vi "Initialize board layout.vi"() -> (0 "Initialized board":refnum<class "Board.lvclass">)   [LabVIEW 2016, in "Chesslib.lvlib" / "Position.lvclass"]
uses:
  Position.lvclass
  Board/Board.lvclass
  typedef/Square.ctl
  typedef/File.ctl
  typedef/Rank.ctl
  typedef/Piece.ctl
  typedef/Color.ctl
  typedef/Piece type.ctl
  Chesslib.lvlib
  Pieces/Piece/Piece.lvclass
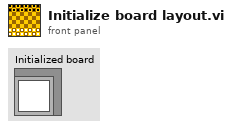
[diagram p1: front panel]
types:
  T1 = typedef "Chesslib.lvlib/Square.ctl" = cluster{"File":T2, "Rank":T3}
  T2 = typedef "Chesslib.lvlib/File.ctl" = enum8{"a", "b", "c", "d", "e", "f", "g", "h"}
  T3 = typedef "Chesslib.lvlib/Rank.ctl" = enum8{"1", "2", "3", "4", "5", "6", "7", "8"}
  T4 = typedef "Chesslib.lvlib/Piece.ctl" = cluster{"Color":T5, "Type":T6}
  T5 = typedef "Chesslib.lvlib/Color.ctl" = enum16{"White", "Black"}
  T6 = typedef "Chesslib.lvlib/Piece type.ctl" = enum16{"Pawn", "Bishop", "Knight", "Rook", "Queen", "King"}
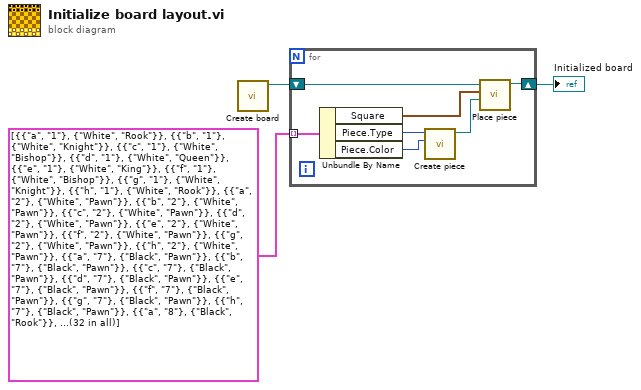
[diagram p0: block diagram]
diagram:
  n1 = call "Create board.vi"() -> ("Empty board"=w2:refnum<class "Board.lvclass">)  [unwired: 11 in]
  n2 = for {
    tunnel: cluster{"Square":T1, "Piece":T4}[] [{"Square"={"File"=enum."a", "Rank"=enum."1"}, "Piece"={"Color"=enum."White", "Type"=enum."Rook"}}, {"Square"={"File"=enum."b", "Rank"=enum."1"}, "Piece"={"Color"=enum."White", "Type"=enum."Knight"}}, {"Square"={"File"=enum."c", "Rank"=enum."1"}, "Piece"={"Color"=enum."White", "Type"=enum."Bishop"}}, {"Square"={"File"=enum."d", "Rank"=enum."1"}, "Piece"={"Color"=enum."White", "Type"=enum."Queen"}}, {"Square"={"File"=enum."e", "Rank"=enum."1"}, "Piece"={"Color"=enum."White", "Type"=enum."King"}}, {"Square"={"File"=enum."f", "Rank"=enum."1"}, "Piece"={"Color"=enum."White", "Type"=enum."Bishop"}}, {"Square"={"File"=enum."g", "Rank"=enum."1"}, "Piece"={"Color"=enum."White", "Type"=enum."Knight"}}, {"Square"={"File"=enum."h", "Rank"=enum."1"}, "Piece"={"Color"=enum."White", "Type"=enum."Rook"}}, {"Square"={"File"=enum."a", "Rank"=enum."2"}, "Piece"={"Color"=enum."White", "Type"=enum."Pawn"}}, {"Square"={"File"=enum."b", "Rank"=enum."2"}, "Piece"={"Color"=enum."White", "Type"=enum."Pawn"}}, {"Square"={"File"=enum."c", "Rank"=enum."2"}, "Piece"={"Color"=enum."White", "Type"=enum."Pawn"}}, {"Square"={"File"=enum."d", "Rank"=enum."2"}, "Piece"={"Color"=enum."White", "Type"=enum."Pawn"}}, {"Square"={"File"=enum."e", "Rank"=enum."2"}, "Piece"={"Color"=enum."White", "Type"=enum."Pawn"}}, {"Square"={"File"=enum."f", "Rank"=enum."2"}, "Piece"={"Color"=enum."White", "Type"=enum."Pawn"}}, {"Square"={"File"=enum."g", "Rank"=enum."2"}, "Piece"={"Color"=enum."White", "Type"=enum."Pawn"}}, {"Square"={"File"=enum."h", "Rank"=enum."2"}, "Piece"={"Color"=enum."White", "Type"=enum."Pawn"}}, {"Square"={"File"=enum."a", "Rank"=enum."7"}, "Piece"={"Color"=enum."Black", "Type"=enum."Pawn"}}, {"Square"={"File"=enum."b", "Rank"=enum."7"}, "Piece"={"Color"=enum."Black", "Type"=enum."Pawn"}}, {"Square"={"File"=enum."c", "Rank"=enum."7"}, "Piece"={"Color"=enum."Black", "Type"=enum."Pawn"}}, {"Square"={"File"=enum."d", "Rank"=enum."7"}, "Piece"={"Color"=enum."Black", "Type"=enum."Pawn"}}, {"Square"={"File"=enum."e", "Rank"=enum."7"}, "Piece"={"Color"=enum."Black", "Type"=enum."Pawn"}}, {"Square"={"File"=enum."f", "Rank"=enum."7"}, "Piece"={"Color"=enum."Black", "Type"=enum."Pawn"}}, {"Square"={"File"=enum."g", "Rank"=enum."7"}, "Piece"={"Color"=enum."Black", "Type"=enum."Pawn"}}, {"Square"={"File"=enum."h", "Rank"=enum."7"}, "Piece"={"Color"=enum."Black", "Type"=enum."Pawn"}}, {"Square"={"File"=enum."a", "Rank"=enum."8"}, "Piece"={"Color"=enum."Black", "Type"=enum."Rook"}}, {"Square"={"File"=enum."b", "Rank"=enum."8"}, "Piece"={"Color"=enum."Black", "Type"=enum."Knight"}}, {"Square"={"File"=enum."c", "Rank"=enum."8"}, "Piece"={"Color"=enum."Black", "Type"=enum."Bishop"}}, {"Square"={"File"=enum."d", "Rank"=enum."8"}, "Piece"={"Color"=enum."Black", "Type"=enum."Queen"}}, {"Square"={"File"=enum."e", "Rank"=enum."8"}, "Piece"={"Color"=enum."Black", "Type"=enum."King"}}, {"Square"={"File"=enum."f", "Rank"=enum."8"}, "Piece"={"Color"=enum."Black", "Type"=enum."Bishop"}}, {"Square"={"File"=enum."g", "Rank"=enum."8"}, "Piece"={"Color"=enum."Black", "Type"=enum."Knight"}}, {"Square"={"File"=enum."h", "Rank"=enum."8"}, "Piece"={"Color"=enum."Black", "Type"=enum."Rook"}}] ("Board layout") -> [w8] mode=indexing
    shift-right: [w9] -> w1
    shift-left: w2 -> [w10]
    n3 = Unbundle By Name(w8) -> ("Square"=w7:T1, "Piece.Type"=w6:T6, "Piece.Color"=w4:T5)
    n4 = call "Create piece.vi"("Piece color"=w4, "Piece type"=w6) -> ("Piece out"=w5:refnum<class "Piece.lvclass">)  [unwired: 9 in]
    n5 = call "Place piece.vi"("Piece"=w5, "Square"=w7, "Board in"=w10) -> ("Board out"=w9:refnum<class "Board.lvclass">)  [unwired: 6 in, 2 out]
  }
  "Initialized board" <- w1
